vi "Write Log File Refnum.vi"(8 "error in (no error)":errorcluster, 10 "Log File Refnum":refnum<file>, 11 "File Sink in":refnum<class "File Sink.lvclass">) -> (0 "error out":errorcluster, 3 "File Sink out":refnum<class "File Sink.lvclass">)   [LabVIEW 2020, in "LV Log.lvlib" / "File Sink.lvclass"]
uses:
  File Sink.lvclass
  File Sink.lvclass/File Sink.ctl
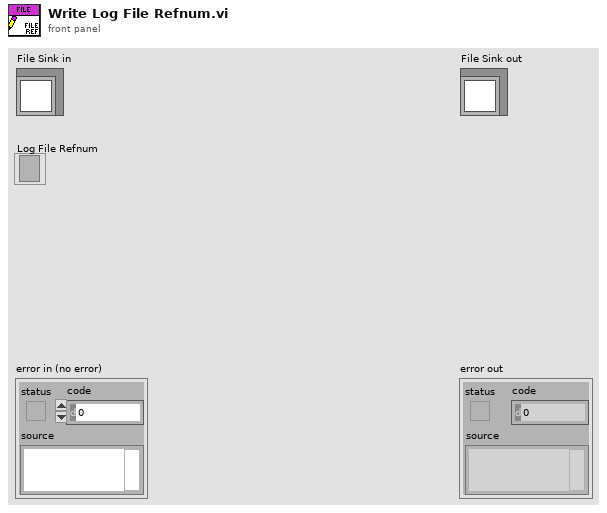
[diagram p1: front panel]
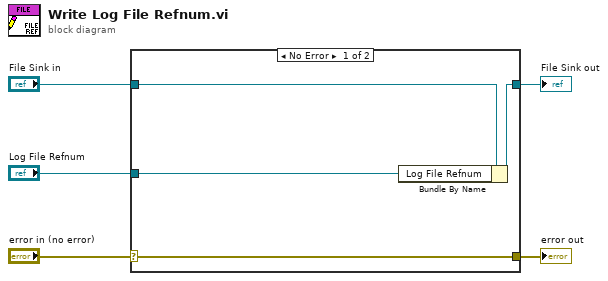
[diagram p0: block diagram]
diagram:
  n1 = case shown="No Error" "error in (no error)" {
    selector: "error in (no error)" -> [w9 w10]
    tunnel: [w9 w10] -> w4
    tunnel: [w7 w11] -> w2
    tunnel: "File Sink in" -> [w8 w11]
    tunnel: "Log File Refnum" -> [w6 _]
    frame No Error {
      n2 = Bundle By Name(cluster=w8, "Log File Refnum"=w6) -> (w7:refnum<class "File Sink.lvclass">)
    }
    frame Error {
    }
  }
  "error out" <- w4
  "File Sink out" <- w2
